vi "VI_RecordingControll_DisableControlls.vi"(7 "Mode":T1, 8 "error in (no error)":errorcluster, 11 "Common Refs":T2) -> (0 "error out":errorcluster)   [LabVIEW 2018]
uses:
  TypeDefs/Refs_Common.ctl
  TypeDefs/TD_Case_RecControll_DisableControlls.ctl
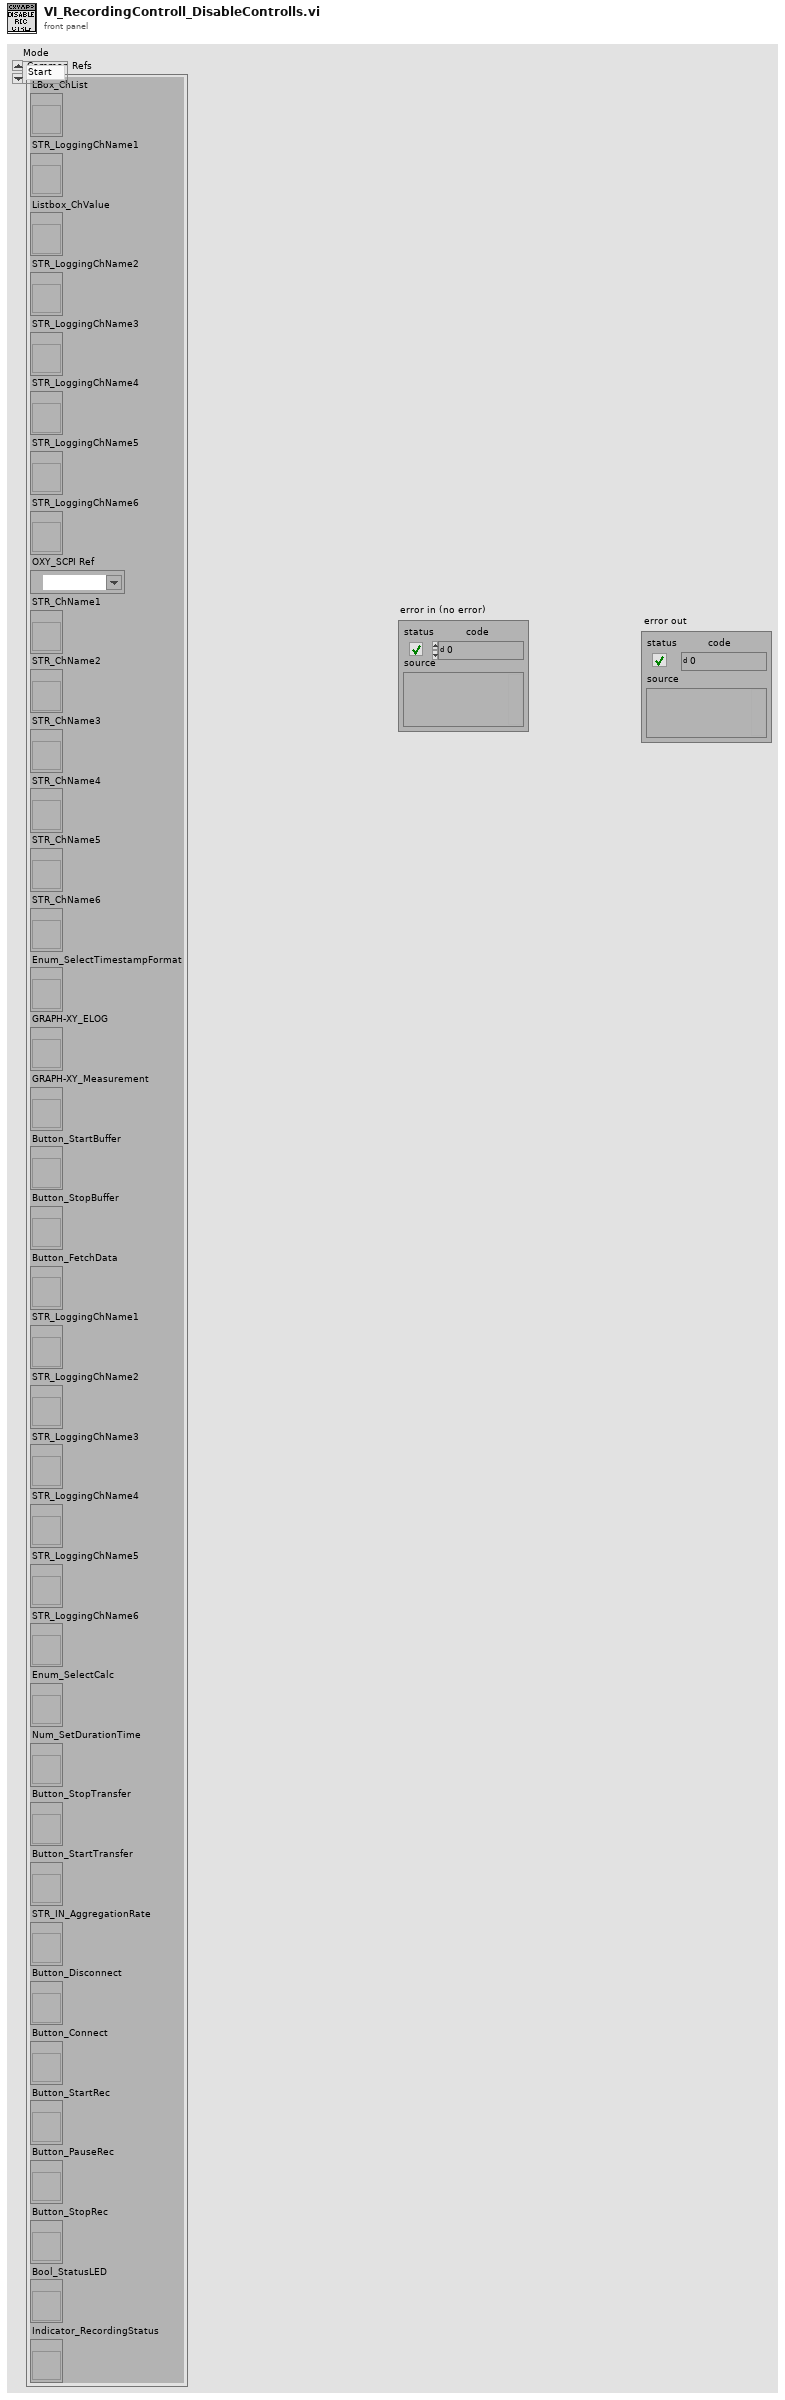
[diagram p1: front panel]
types:
  T1 = typedef "TD_Case_RecControll_DisableControlls.ctl" = enum16{"Start", "Pause", "Stop"}
  T2 = typedef "Refs_Common.ctl" = cluster{"LBox_ChList":refnum<vi>, "STR_LoggingChName1":refnum<vi>, "Listbox_ChValue":refnum<vi>, "STR_LoggingChName2":refnum<vi>, "STR_LoggingChName3":refnum<vi>, "STR_LoggingChName4":refnum<vi>, "STR_LoggingChName5":refnum<vi>, "STR_LoggingChName6":refnum<vi>, "OXY_SCPI Ref":refnum<visa-resource-name>, "STR_ChName1":refnum<vi>, "STR_ChName2":refnum<vi>, "STR_ChName3":refnum<vi>, "STR_ChName4":refnum<vi>, "STR_ChName5":refnum<vi>, "STR_ChName6":refnum<vi>, "Enum_SelectTimestampFormat":refnum<vi>, "GRAPH-XY_ELOG":refnum<vi>, "GRAPH-XY_Measurement":refnum<vi>, "Button_StartBuffer":refnum<vi>, "Button_StopBuffer":refnum<vi>, "Button_FetchData":refnum<vi>, "STR_LoggingChName1":refnum<vi>, "STR_LoggingChName2":refnum<vi>, "STR_LoggingChName3":refnum<vi>, "STR_LoggingChName4":refnum<vi>, "STR_LoggingChName5":refnum<vi>, "STR_LoggingChName6":refnum<vi>, "Enum_SelectCalc":refnum<vi>, "Num_SetDurationTime":refnum<vi>, "Button_StopTransfer":refnum<vi>, "Button_StartTransfer":refnum<vi>, "STR_IN_AggregationRate":refnum<vi>, "Button_Disconnect":refnum<vi>, "Button_Connect":refnum<vi>, "Button_StartRec":refnum<vi>, "Button_PauseRec":refnum<vi>, "Button_StopRec":refnum<vi>, "Bool_StatusLED":refnum<vi>, "Indicator_RecordingStatus":refnum<vi>}
  T3 = enum8{"Enabled", "Disabled", "Disabled and Grayed Out"}
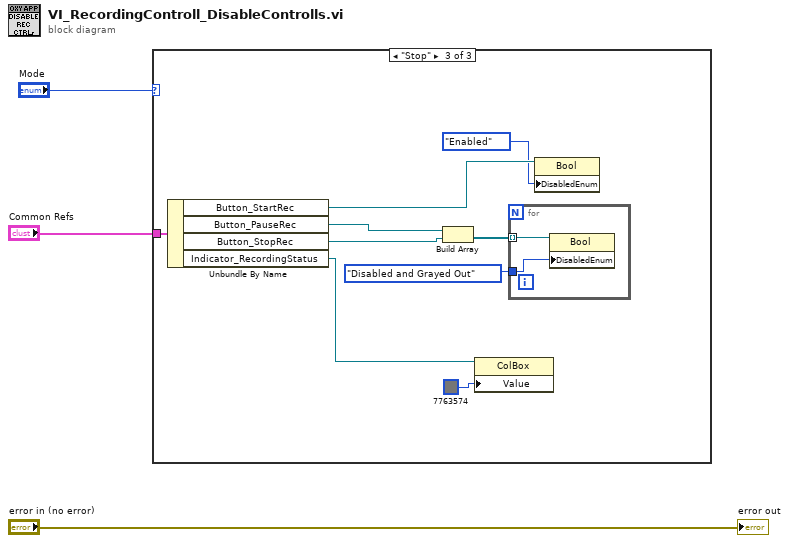
[diagram p0: block diagram]
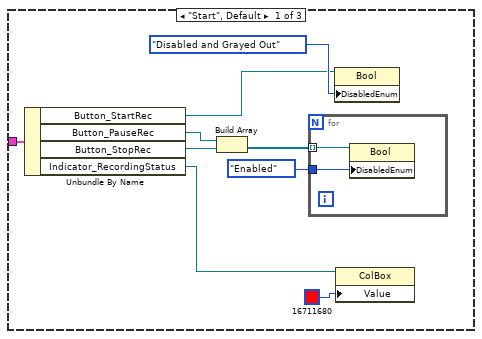
[diagram p2: hidden frame]
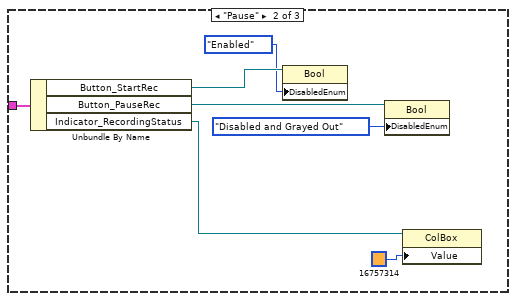
[diagram p3: hidden frame]
diagram:
  n1 = case shown="\"Stop\"" "Mode" {
    tunnel: "Common Refs" -> [w6 w17 w24]
    frame "Start", Default {
      n2 = Unbundle By Name(w6) -> ("Button_StartRec"=w11:refnum<vi>, "Button_PauseRec"=w7:refnum<vi>, "Button_StopRec"=w8:refnum<vi>, "Indicator_RecordingStatus"=w5:refnum<vi>)
      n3 = Build Array(w7, w8) -> (w9:refnum<vi>[])
      n4 = for {
        tunnel: w9 -> [w14] mode=indexing
        tunnel: T3."Enabled" ("Disabled") -> [w13]
        n5 = property class="Bool"(reference=w14, "DisabledEnum"=w13) -> ()  [unwired: 1 in, 2 out]
      }
      n6 = property class="Bool"(reference=w11, "DisabledEnum"=T3."Disabled and Grayed Out" ("Disabled")) -> ()  [unwired: 1 in, 2 out]
      n7 = property class="ColBox"(reference=w5, "Value"=u32 16711680 ("Color Box")) -> ()  [unwired: 1 in, 2 out]
    }
    frame "Pause" {
      n8 = Unbundle By Name(w17) -> ("Button_StartRec"=w20:refnum<vi>, "Button_PauseRec"=w18:refnum<vi>, "Indicator_RecordingStatus"=w15:refnum<vi>)
      n9 = property class="Bool"(reference=w20, "DisabledEnum"=T3."Enabled" ("Disabled")) -> ()  [unwired: 1 in, 2 out]
      n10 = property class="Bool"(reference=w18, "DisabledEnum"=T3."Disabled and Grayed Out" ("Disabled")) -> ()  [unwired: 1 in, 2 out]
      n11 = property class="ColBox"(reference=w15, "Value"=u32 16757314 ("Color Box")) -> ()  [unwired: 1 in, 2 out]
    }
    frame "Stop" {
      n12 = Unbundle By Name(w24) -> ("Button_StartRec"=w26:refnum<vi>, "Button_PauseRec"=w30:refnum<vi>, "Button_StopRec"=w29:refnum<vi>, "Indicator_RecordingStatus"=w22:refnum<vi>)
      n13 = Build Array(w30, w29) -> (w28:refnum<vi>[])
      n14 = property class="ColBox"(reference=w22, "Value"=u32 7763574 ("Color Box")) -> ()  [unwired: 1 in, 2 out]
      n15 = for {
        tunnel: w28 -> [w32] mode=indexing
        tunnel: T3."Disabled and Grayed Out" ("Disabled") -> [w31]
        n16 = property class="Bool"(reference=w32, "DisabledEnum"=w31) -> ()  [unwired: 1 in, 2 out]
      }
      n17 = property class="Bool"(reference=w26, "DisabledEnum"=T3."Enabled" ("Disabled")) -> ()  [unwired: 1 in, 2 out]
    }
  }
  "error out" <- "error in (no error)"
